vi "PCO_GetFlimModulationParameter.vi"(8 "error in (no error)":errorcluster {"code" format="%x"}, 11 "ph":u64) -> (0 "error out":errorcluster {"code" format="%x"}, 1 "wSourceSelect":u16(ring) items=["intern", "extern"], 2 "ErrorMessage":i32 format="%x", 3 "ph out":u64, 5 "wOutputWaveform":u16(ring) items=["none", "sine wave", "square wave"])   [LabVIEW 2019, in "SDK.lvlib" / "SpecialCommandsFlim.lvlib"]
doc: "<b>Description:</b>\nThis function can be used to query the current modulation signal settings of the pco.flim.\n\n<b>Supported camera type</b>\npco.flim\n\n<b>Descriptor dependency:</b>\nNone"
uses:
  SpecialCommandsFlim.lvlib
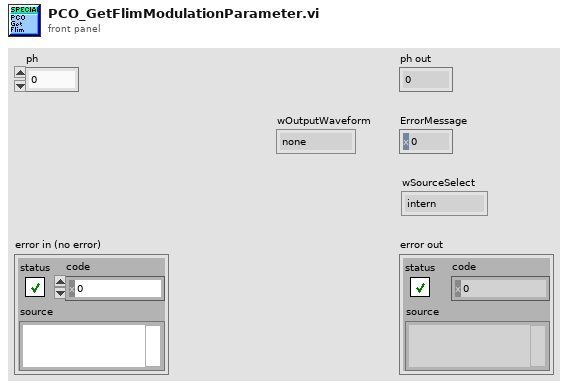
[diagram p1: front panel]
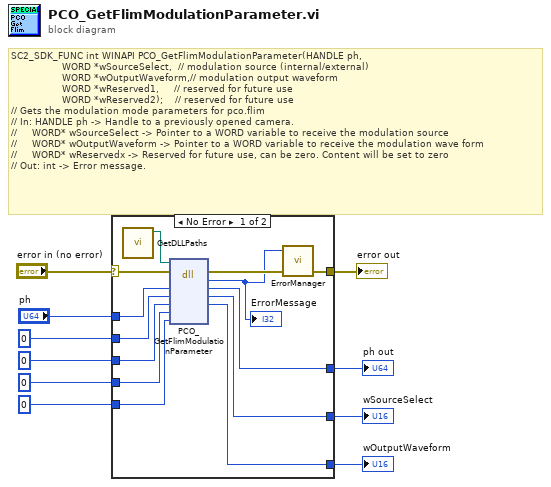
[diagram p0: block diagram]
diagram:
  # "SC2_SDK_FUNC int WINAPI PCO_GetFlimModulationParameter(HANDLE ph, \n                 WORD *wSourceSelect,  // modulation source (internal/external)\n                 WORD *wOutputWaveform,// modulation output waveform\n                 WORD *wReserved1,     // reserved for future use\n                 WORD *wReserved2);    // reserved for future use\n// Gets the modulation mode parameters for pco.flim\n// In: HANDLE ph -> Handle to a previously opened camera.\n//     WORD* wSourceSelect -> Pointer to a WORD variable to receive the modulation source\n//     WORD* wOutputWaveform -> Pointer to a WORD variable to receive the modulation wave form\n//     WORD* wReservedx -> Reserved for future use, can be zero. Content will be set to zero\n// Out: int -> Error message."
  n1 = case shown="No Error" "error in (no error)" {
    selector: "error in (no error)" -> [w15 w27]
    tunnel: "ph" -> [w23 w26]
    tunnel: [w22 w26] -> w9
    tunnel: u16 0 ("wSourceSelect") -> [w21 w25]
    tunnel: [w20 w25] -> w7
    tunnel: u16 0 ("wOutputWaveform") -> [w19 w24]
    tunnel: [w18 w24] -> w5
    tunnel: u16 0 ("wReserved1") -> [w17 _]
    tunnel: u16 0 ("wReserved2") -> [w16 _]
    tunnel: [w14 w27] -> w2
    frame No Error {
      n2 = call "GetDLLPaths.vi"() -> ("SC2_Cam_Path"=w11:path)  [unwired: 8 in, 3 out]
      n3 = dll-call lib="?" fn="PCO_GetFlimModulationParameter"(path in=w11, error in=w15, "ph"=w23, "wSourceSelect"=w21, "wOutputWaveform"=w19, "wReserved1"=w17, "wReserved2"=w16) -> (error out=w13:errorcluster, "return type"=w12:i32, "ph"=w22:u64, "wSourceSelect"=w20:u16, "wOutputWaveform"=w18:u16)  [unwired: 3 in, 1 out]
      "ErrorMessage" <- w12
      n4 = call "ErrorManager.vi"("error in (no error)"=w13, "error code"=w12) -> ("error out"=w14:errorcluster)  [unwired: 2 in, 1 out]
    }
    frame Error {
    }
  }
  "ph out" <- w9
  "wSourceSelect" <- w7
  "wOutputWaveform" <- w5
  "error out" <- w2
